vi "Replace EmptyCell Mark.vi"(8 "error in (no error)":errorcluster, 9 "EmptyCellToken(^[\\/]$)":string="^[\\/]$", 11 "CfgTable in":string[][](array[string])) -> (0 "error out":errorcluster, 3 "data 2":string[][](array[string]))   [LabVIEW 2017, in "ClusterCfgTable.lvlib"]
uses:
  ClusterCfgTable.lvlib
  <userlib>/_OpenG.lib/string/string.llb/Trim Whitespace (String)__ogtk.vi
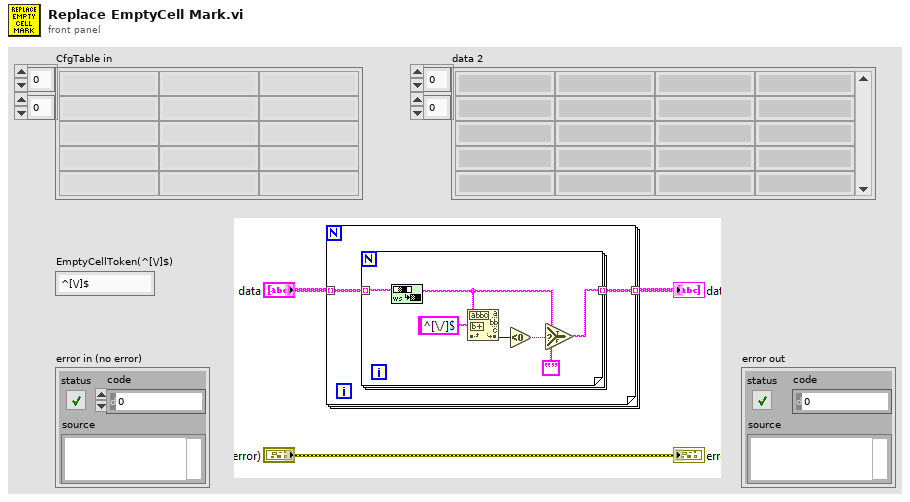
[diagram p1: front panel]
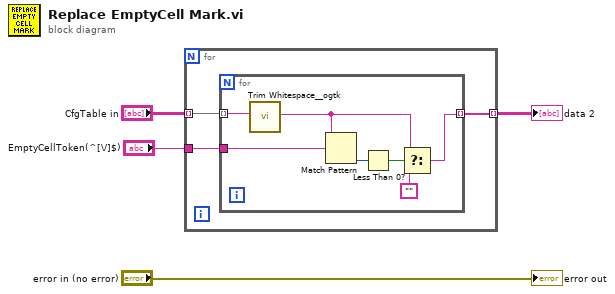
[diagram p0: block diagram]
diagram:
  n1 = for {
    tunnel: "CfgTable in" -> [w6] mode=indexing
    tunnel: [w7] -> w3 mode=indexing
    tunnel: "EmptyCellToken(^[\\/]$)" -> [w5]
    n2 = for {
      tunnel: [w9] -> w7 mode=indexing
      tunnel: w6 -> [w14] mode=indexing
      tunnel: w5 -> [w8]
      n3 = call-poly <userlib>:"Trim Whitespace__ogtk.vi"("String in"=w14) -> ("String out"=w11:string)  [unwired: 6 in]
      n4 = Match Pattern(string=w11, regular expression=w8) -> (offset past match=w13:i32)  [unwired: 1 in, 3 out]
      n5 = Less Than 0?(x=w13) -> (x < 0?=w12:bool)
      n6 = Select(t=w11, s=w12, f="") -> (s? t:f=w9:string)
    }
  }
  "data 2" <- w3
  "error out" <- "error in (no error)"
